vi "tt20_make_counter.vi"(8 "error in (no error)":errorcluster, 11 "tt20 in":refnum<class "tt20.lvclass">) -> (0 "error out":errorcluster, 3 "tt20 out":refnum<class "tt20.lvclass">)   [LabVIEW 2015, in "tt20.lvclass"]
uses:
  tt20.lvclass
  tt20.lvclass/tt20.ctl
  C:/Users/MX-Microscope/Documents/LabVIEW Data/lvoop_campus_2018/Detector_Class/Swabian/time_tagger_vis/TTCSharp32.dll
  time_tagger_vis/TTCSharp32.dll
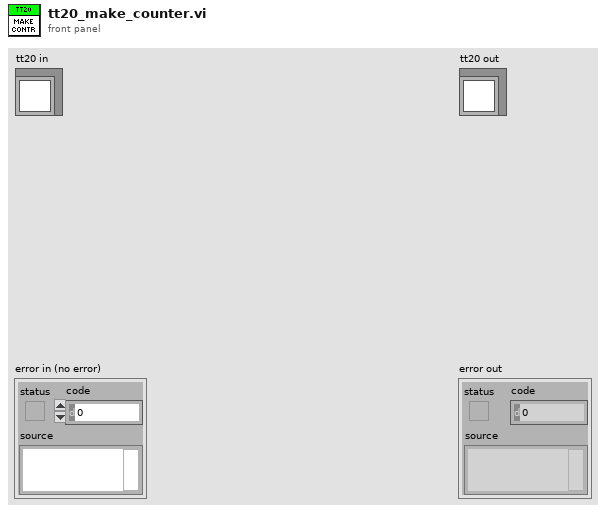
[diagram p1: front panel]
types:
  T1 = typedef "tt20_acq_mode_tdef.ctl" = enum16{"T2", "T3"}
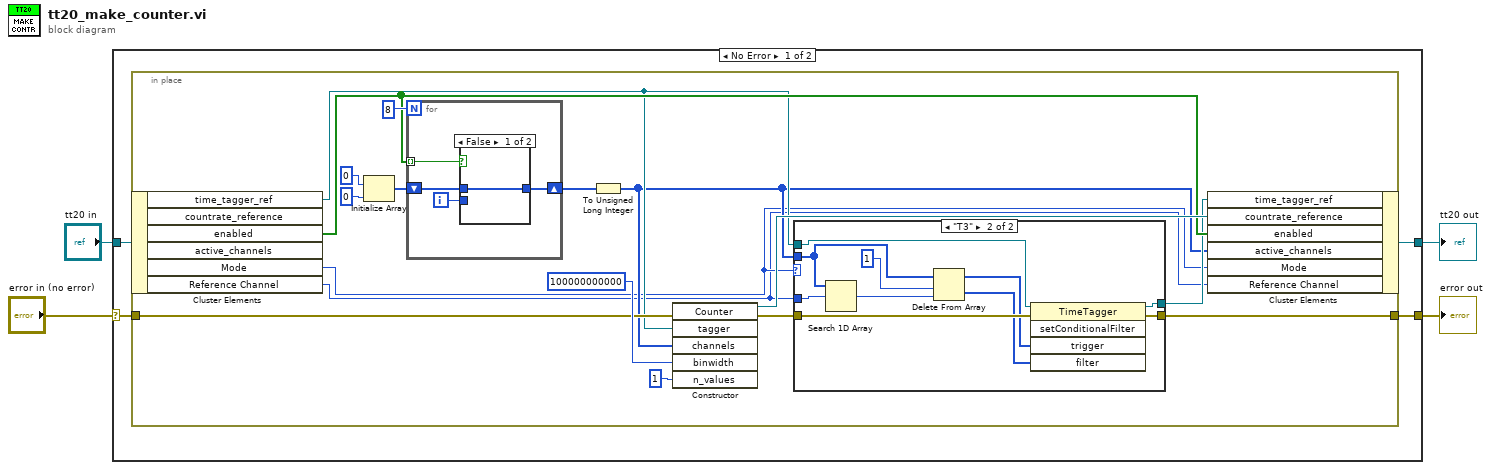
[diagram p0: block diagram]
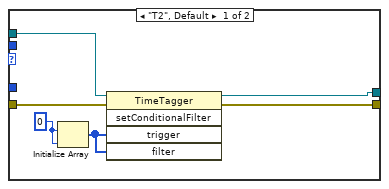
[diagram p2: hidden frame]
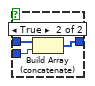
[diagram p3: hidden frame]
diagram:
  n1 = case shown="No Error" "error in (no error)" {
    selector: "error in (no error)" -> [w8 w51]
    tunnel: [w7 w51] -> w3
    tunnel: [w5 w50] -> w1
    tunnel: "tt20 in" -> [w6 w50]
    frame No Error {
      n2 = in-place {
        in-place-border: w8 -> [w22]
        in-place-border: [w13] -> w7
        n3 = in-place-cluster #1(w6) -> ("time_tagger_ref"=w15:refnum<k24>, "enabled"=w20:bool[], "Mode"=w10:T1, "Reference Channel"=w9:u8)  [unwired: 2 out]
        n4 = Initialize Array(0 ("element"), 0 ("dimension size")) -> (w19:i32[])
        n5 = for {
          N: 8 -> [_]
          tunnel: w20 -> [w45] mode=indexing
          shift-right: [w43] -> w16
          shift-left: w19 -> [w42]
          i -> [w44]
          n6 = case shown="False" w45 {
            tunnel: w44 -> [_ w49]
            tunnel: [w46 w48] -> w43
            tunnel: w42 -> [w46 w47]
            frame False {
            }
            frame True {
              n7 = Build Array (concatenate)(w47, w49) -> (w48:i32[])
            }
          }
        }
        n8 = To Unsigned Long Integer(number=w16) -> (unsigned 32bit integer=w11:u32[])
        n9 = constructor class="Counter"(error in=w22, "tagger"=w15, "channels"=w11, "binwidth"=i64 100000000000, "n_values"=1) -> (reference out=w23:refnum<k24>, error out=w14:errorcluster)  [unwired: 2 in, 5 out]
        n10 = case shown="\"T3\"" w10 {
          tunnel: w14 -> [w31 w41]
          tunnel: [w30 w40] -> w13
          tunnel: w15 -> [w29 w39]
          tunnel: [w28 w38] -> w12
          tunnel: w11 -> [_ w36]
          tunnel: w9 -> [_ w37]
          frame "T2", Default {
            w27 = 0 ("dimension size")
            n11 = Initialize Array(w27, w27) -> (w26:i32[])
            n12 = invoke class="TimeTagger" method="setConditionalFilter"(reference=w29, error in=w31, "trigger"=w26, "filter"=w26) -> (reference out=w28:refnum<k24>, error out=w30:errorcluster)  [unwired: 1 in, 3 out]
          }
          frame "T3" {
            n13 = Search 1D Array(1D array=w36, element=w37) -> (index of element=w35:i32)  [unwired: 1 in]
            n14 = Delete From Array(array=w36, length=1, index=w35) -> (deleted portion=w32:u32[], array with subset deleted=w33:u32[])
            n15 = invoke class="TimeTagger" method="setConditionalFilter"(reference=w39, error in=w41, "trigger"=w33, "filter"=w32) -> (reference out=w38:refnum<k24>, error out=w40:errorcluster)  [unwired: 1 in, 3 out]
          }
        }
        n16 = in-place-cluster #1("time_tagger_ref"=w12, "countrate_reference"=w23, "enabled"=w20, "active_channels"=w11, "Mode"=w10, "Reference Channel"=w9) -> (w5:refnum<class "tt20.lvclass">)
      }
    }
    frame Error {
    }
  }
  "error out" <- w3
  "tt20 out" <- w1
